vi "Main.vi"(8 "error in":errorcluster, 11 "Head_ScopeSim in":refnum<class "Head_ScopeSim.lvclass">) -> (0 "error out":errorcluster, 3 "Head_ScopeSim out":refnum<class "Head_ScopeSim.lvclass">)   [LabVIEW 2019, in "Head_ScopeSim.lvclass"]
doc: "The <b>Queued Message Handler</b> of the Worker that owns this VI."
uses:
  Head_ScopeSim.lvclass
  C:/Program Files (x86)/National Instruments/LabVIEW 2019/vi.lib/addons/_Workers/Library/Classes/Worker/Worker.lvclass
  Head_ScopeSim.lvclass/Head_ScopeSim.ctl
  Initialization Data.ctl
  Response Cases.ctl
  rql_Create gRPC Server.ctl
  gRPC Server/gRPC Server/rwr_Create gRPC Server.ctl
  rql_Destroy gRPC Server.ctl
  Scope Simulator/rqp_Scope Configuration.ctl
  Scope Simulator/rqp_Run Scope.ctl
  gRPC Server/gRPC Server/rqp_Msg_ToClient_2.ctl
  Generated_server/RPC Messages/w4lvgrpc_Msg_ToClient_2.ctl
  gRPC Server/gRPC Server/rqp_Msg_ToClient_3.ctl
  Generated_server/RPC Messages/w4lvgrpc_Msg_ToClient_3.ctl
  Generated_server/RPC Messages/w4lvgrpc_State.ctl
  <vilib>/addons/_Workers/Library/Classes/Message Queue/Message Queue.lvclass
  Scope Simulator/Scope Simulator.lvclass
  gRPC Server/gRPC Server/gRPC Server.lvclass
  Generated_server/Generated_server.lvlib
panel:
  out "Client ID":u64
  out "Client Connected":bool
  out "Listening Port":i32
  out "Server Listening":bool
  in  "Server Address":string="localhost:50070"
  in  "Destroy gRPC Server":bool
  in  "Create gRPC Server":bool
  # "Workers <-> Python gRPC Example"
  # "Scope Simulator"
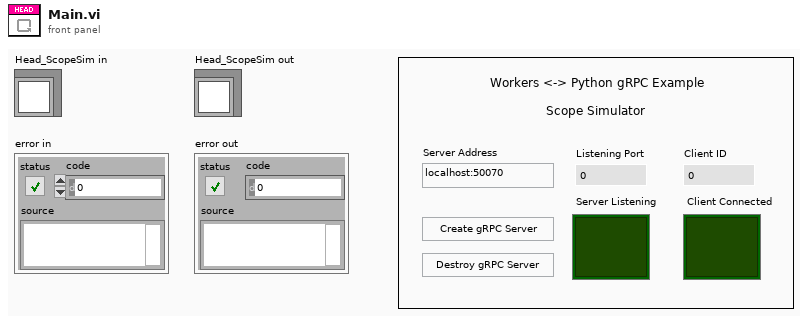
[diagram p1: front panel]
types:
  T1 = typedef "Head_ScopeSim.lvclass/Initialization Data.ctl" = cluster{"Response Cases":T2}
  T2 = typedef "Head_ScopeSim.lvclass/Response Cases.ctl" = cluster{"Placeholder - Can be deleted":string}
  T3 = typedef "Head_ScopeSim.lvclass/rql_Create gRPC Server.ctl" = cluster{"String":string}
  T4 = typedef "gRPC Server (scope.proto).lvlib/gRPC Server.lvclass/rwr_Create gRPC Server.ctl" = cluster{"Server Key File (.key)":path, "Server Certificate File (.crt)":path, "Server Address":string}
  T5 = typedef "Head_ScopeSim.lvclass/rql_Destroy gRPC Server.ctl" = cluster{"String":string}
  T6 = typedef "Scope Simulator.lvclass/rqp_Scope Configuration.ctl" = cluster{"physical_channel":string, "sample_rate_hz":dbl, "samples_per_read":i32}
  T7 = typedef "Scope Simulator.lvclass/rqp_Run Scope.ctl" = cluster{"Run Scope ?":bool}
  T8 = typedef "gRPC Server (scope.proto).lvlib/gRPC Server.lvclass/rqp_Msg_ToClient_2.ctl" = cluster{"w4lvgrpc_Msg_ToClient_2":T9}
  T9 = typedef "Generated_server.lvlib/w4lvgrpc_Msg_ToClient_2.ctl" = cluster{"y":dbl[], "dt":dbl, "t0":dbl, "label":string, "acquisitions":i32}
  T10 = typedef "gRPC Server (scope.proto).lvlib/gRPC Server.lvclass/rqp_Msg_ToClient_3.ctl" = cluster{"w4lvgrpc_Msg_ToClient_3":T11}
  T11 = typedef "Generated_server.lvlib/w4lvgrpc_Msg_ToClient_3.ctl" = cluster{"state":T12}
  T12 = typedef "Generated_server.lvlib/w4lvgrpc_State.ctl" = enum32{"STOPPED", "RUNNING", "ERROR"}
  T13 = typedef "gRPC Server (scope.proto).lvlib/gRPC Server.lvclass/rwr_Create gRPC Server Reply.ctl" = cluster{"Listening Port":i32}
  T14 = typedef "gRPC Server (scope.proto).lvlib/gRPC Server.lvclass/rsp_Connection Notify.ctl" = cluster{"gRPC ID":T15, "Connected?":bool}
  T15 = typedef "grpc-lvsupport-release.lvlib/grpcId.ctl" = u64
  T16 = typedef "gRPC Server (scope.proto).lvlib/gRPC Server.lvclass/rsp_Server Error.ctl" = errorcluster
  T17 = typedef "gRPC Server (scope.proto).lvlib/gRPC Server.lvclass/rsp_Msg_ToServer_1.ctl" = cluster{"w4lvgrpc_Msg_ToServer_1":T18}
  T18 = typedef "Generated_server.lvlib/w4lvgrpc_Msg_ToServer_1.ctl" = cluster{"physical_channel":string, "sample_rate_hz":dbl, "samples_per_read":i32}
  T19 = typedef "gRPC Server (scope.proto).lvlib/gRPC Server.lvclass/rsp_Msg_ToServer_2.ctl" = cluster{"w4lvgrpc_Msg_ToServer_2":T20}
  T20 = typedef "Generated_server.lvlib/w4lvgrpc_Msg_ToServer_2.ctl" = cluster{"run":bool}
  T21 = typedef "Scope Simulator.lvclass/rsp_Generated Waveform.ctl" = cluster{"y":dbl[], "Acquisitions":i32}
  T22 = typedef "Scope Simulator.lvclass/rsp_Scope Status.ctl" = enum32{"STOPPED", "RUNNING", "ERROR"}
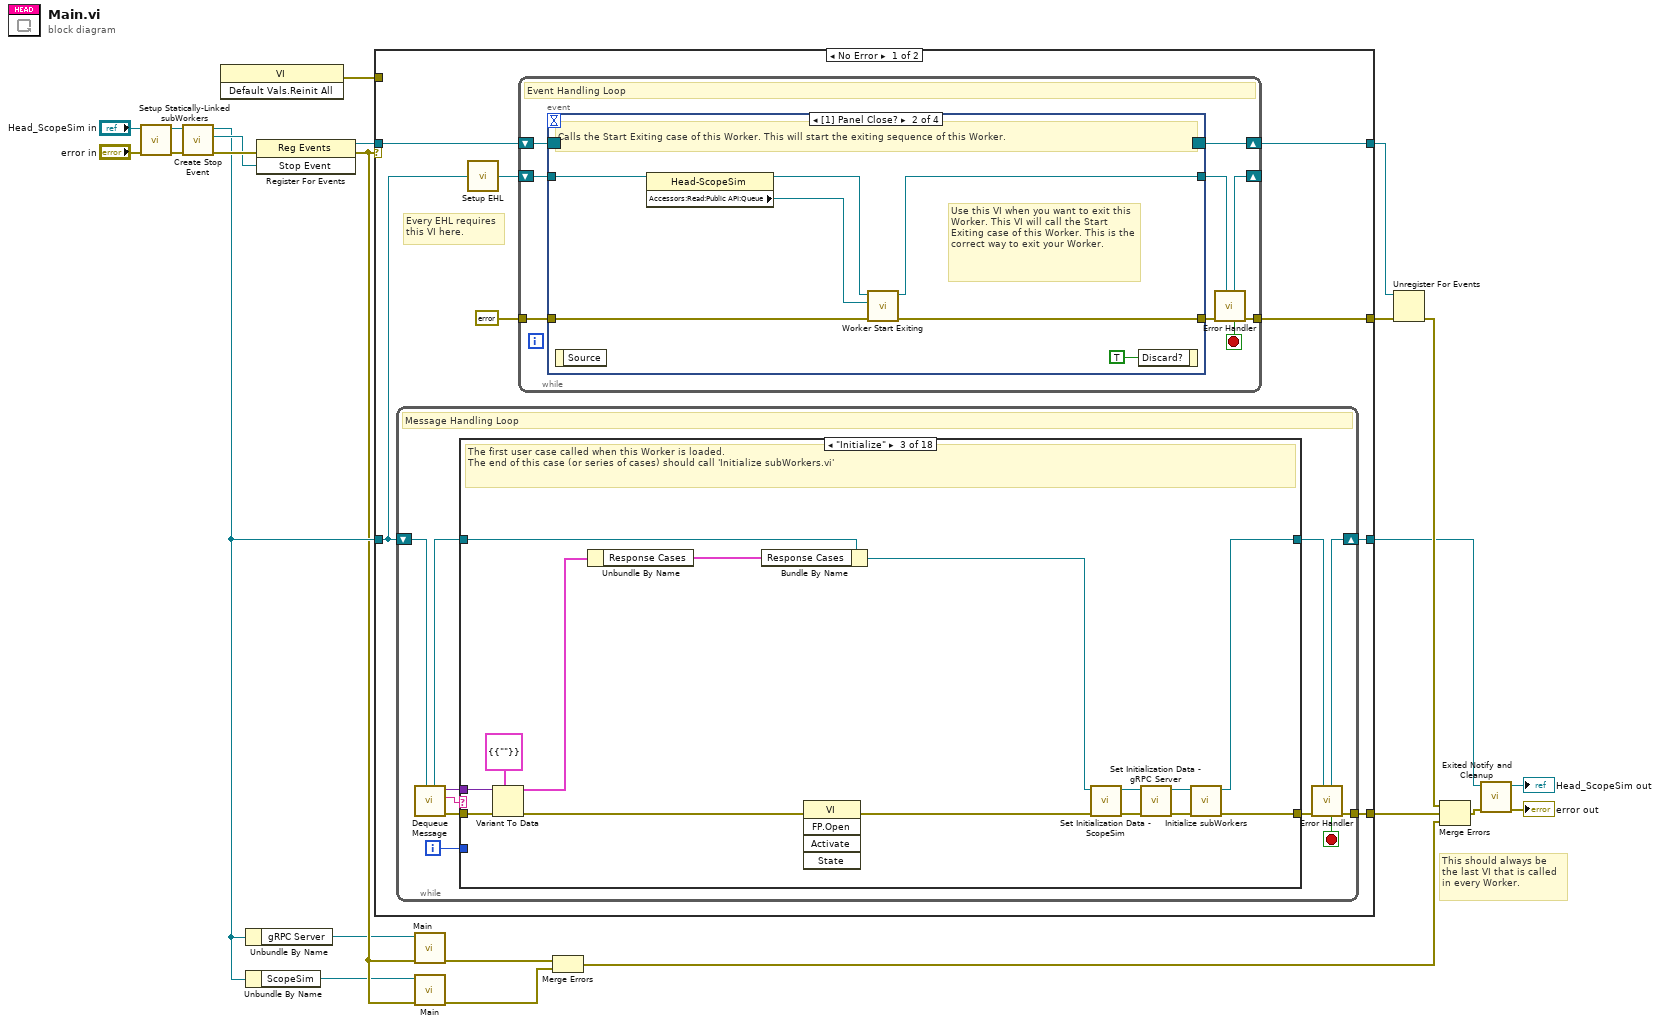
[diagram p0: block diagram]
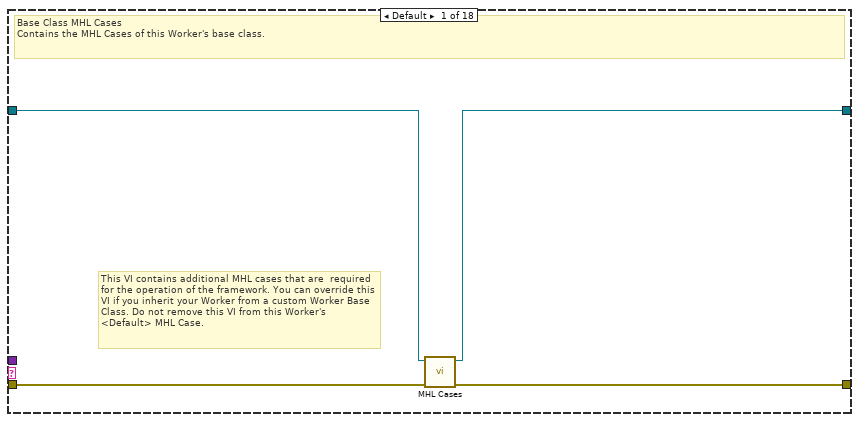
[diagram p2: hidden frame]
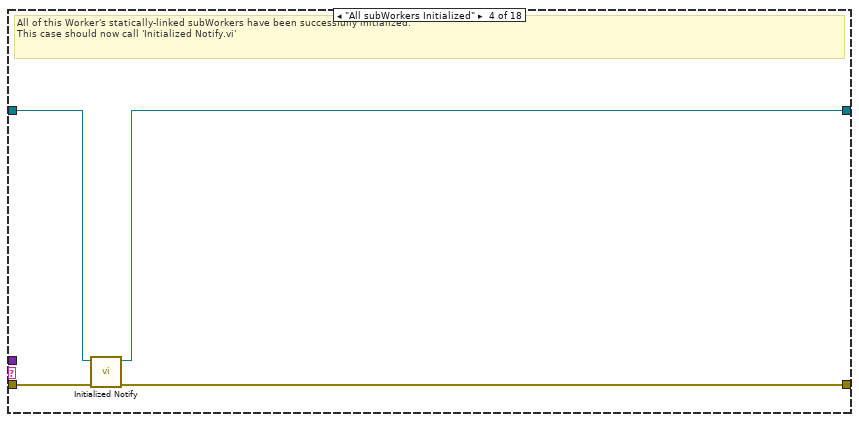
[diagram p4: hidden frame]
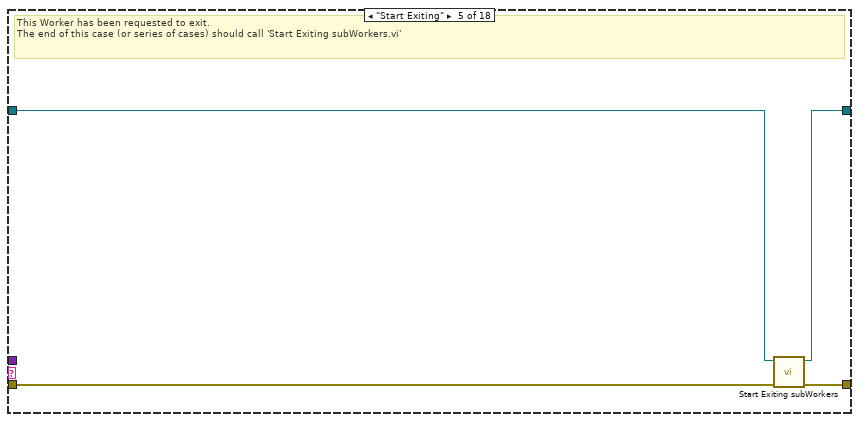
[diagram p5: hidden frame]
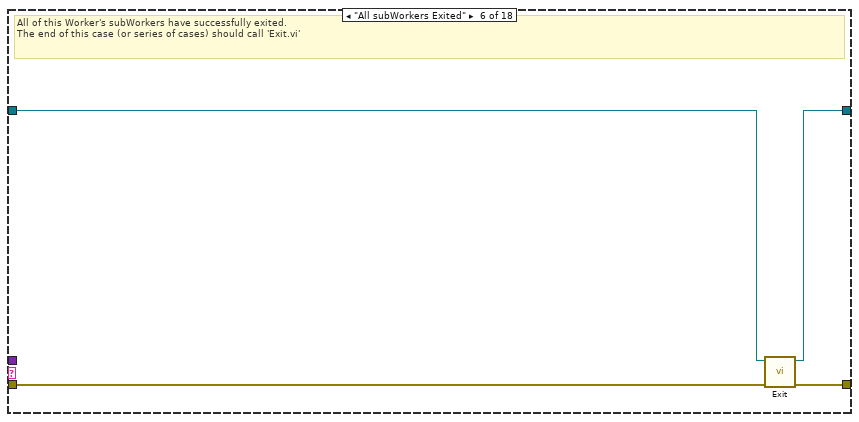
[diagram p6: hidden frame]
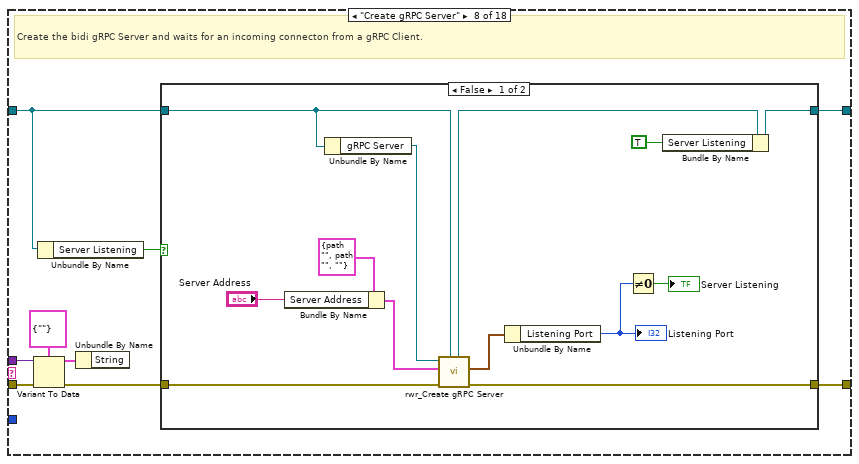
[diagram p8: hidden frame]
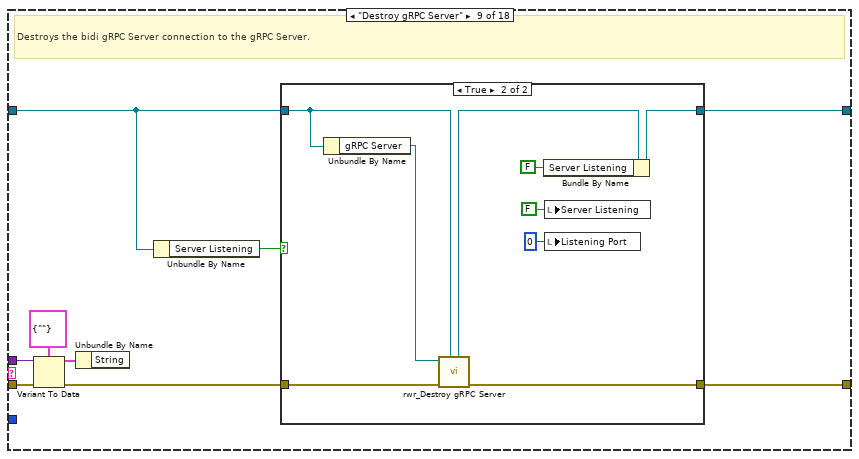
[diagram p10: hidden frame]
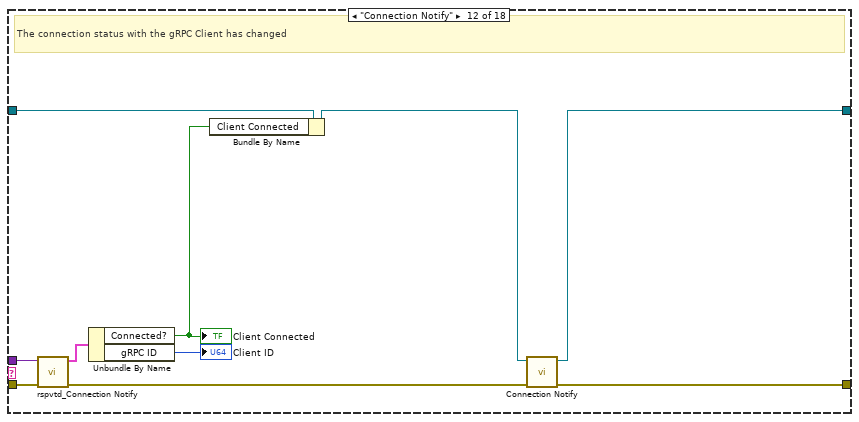
[diagram p14: hidden frame]
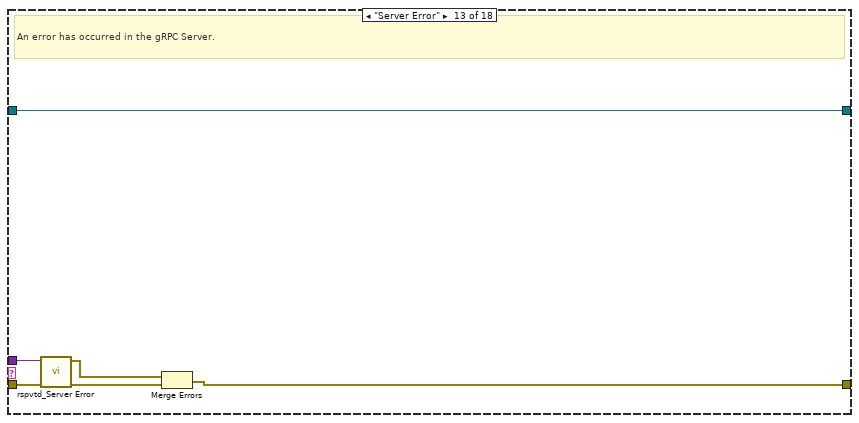
[diagram p15: hidden frame]
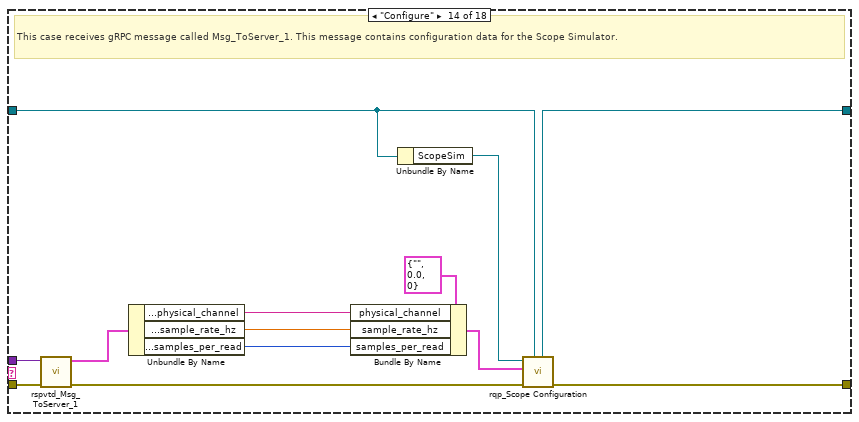
[diagram p16: hidden frame]
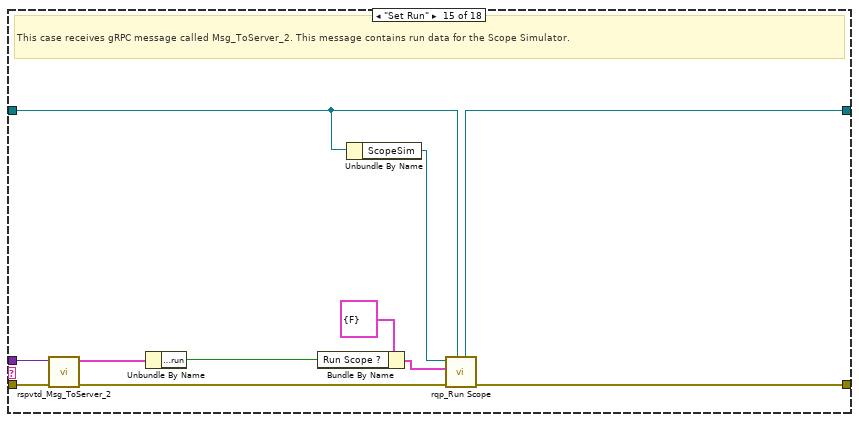
[diagram p17: hidden frame]
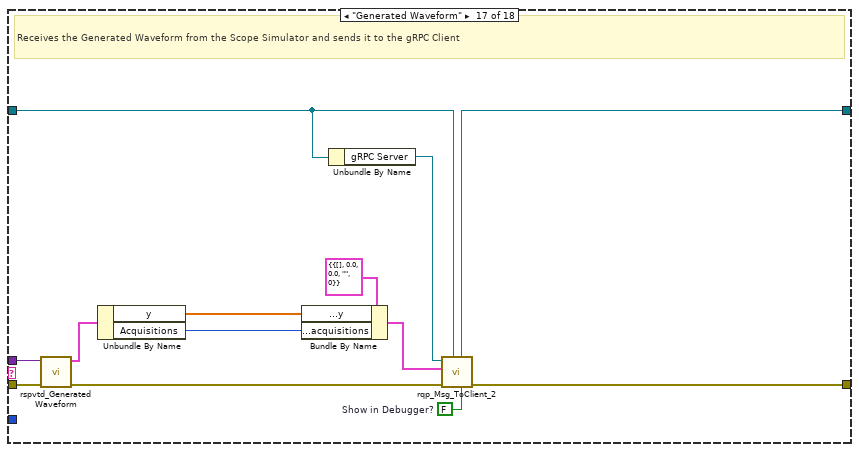
[diagram p19: hidden frame]
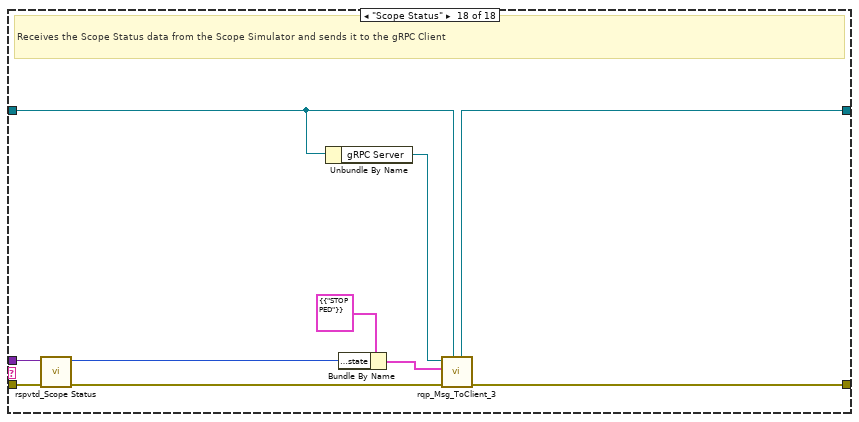
[diagram p20: hidden frame]
diagram:
  # "This should always be the last VI that is called in every Worker."
  n1 = call "Setup Statically-Linked subWorkers.vi"("error in"="error in", "Head_ScopeSim in"="Head_ScopeSim in") -> ("error out"=w9:errorcluster, "Head_ScopeSim out"=w7:refnum<class "Head_ScopeSim.lvclass">)  [unwired: 8 in]
  n2 = call-dynamic "Create Stop Event.vi"("error in"=w9, "Worker"=w7) -> ("error out"=w18:errorcluster, "Stop Event"=w15:refnum<user-event>, "Worker out"=w12:refnum<class "Head_ScopeSim.lvclass">)  [unwired: 7 in]
  n3 = invoke class="VI" method="Default Vals.Reinit All"() -> (error out=w3:errorcluster)  [unwired: 3 in, 2 out]
  n4 = Unbundle By Name(w12) -> ("gRPC Server"=w4:refnum<class "gRPC Server.lvclass">)
  n5 = Unbundle By Name(w12) -> ("ScopeSim"=w1:refnum<class "Scope Simulator.lvclass">)
  n6 = register-events(error in=w18, w15) -> (reference out=w17:refnum<event-registration>, error out=w10:errorcluster)  [unwired: 1 in]
  n7 = case shown="No Error" w10 {
    tunnel: w12 -> [w26 w221]
    tunnel: [w24 w222] -> w16
    tunnel: w17 -> [w31 w223]
    tunnel: [w28 w224] -> w22
    tunnel: [w30 w223] -> w21
    tunnel: [w25 w220] -> w19
    selector: w10 -> [_ w224]
    tunnel: w3 -> [_ _]
    frame No Error {
      # "Every EHL requires\nthis VI here."
      n8 = while {
        shift-right: [w40] -> w25
        shift-left: w26 -> [w42]
        tunnel: [w41] -> w24
        i -> [w33]
        stop <- w34 stop-if-true
        # "Message Handling Loop"
        n9 = call-dynamic "Dequeue Message.vi"("Worker"=w42) -> ("error out"=w39:errorcluster, "Case out"=w35:string, "Data out"=w32:variant, "Worker out"=w37:refnum<class "Head_ScopeSim.lvclass">)  [unwired: 6 in, 1 out]
        n10 = case "Worker MHL Case Structure (DO NOT CHANGE LABEL NAME)" shown="\"Initialize\"" w35 {
          tunnel: w39 -> [w46 w47 w61 w66 w68 w75 w77 w86 w110 w123 w125 w135 w141 w154 w165 w167 w180 w190]
          tunnel: [w45 w47 w63 w64 w71 w74 w77 w81 w105 w123 w125 w128 w137 w150 w161 w167 w177 w187] -> w38
          tunnel: w37 -> [w44 w48 w60 w67 w69 w73 w76 w79 w103 w122 w124 w134 w140 w148 w159 w166 w175 w185]
          tunnel: [w43 w48 w62 w65 w70 w72 w76 w80 w104 w122 w124 w130 w140 w149 w160 w166 w176 w186] -> w36
          tunnel: w33 -> [_ _ _ _ _ _ _ _ _ _ _ _ _ _ _ _ _ _]
          tunnel: w32 -> [_ _ w59 _ _ _ _ w83 w107 _ _ w133 w138 w152 w164 _ w178 w188]
          frame Default {
            # "This VI contains additional MHL cases that are  required for the operation of the framework. You can override this VI if you inherit your Worker from a custom Worker Base Class. Do not remove this VI from this Worker's <Default> MHL Case."
            # "Base Class MHL Cases\nContains the MHL Cases of this Worker's base class."
            n11 = call-dynamic "MHL Cases.vi"("error in"=w46, "Worker in"=w44) -> ("error out"=w45:errorcluster, "Worker out"=w43:refnum<class "Head_ScopeSim.lvclass">)  [unwired: 8 in]
          }
          frame "------------ FRAMEWORK CASES -----------" {
            # "Start of Workers Framework Cases"
          }
          frame "Initialize" {
            # "The first user case called when this Worker is loaded.\nThe end of this case (or series of cases) should call 'Initialize subWorkers.vi'"
            n12 = Variant To Data(error in=w61, type=T1 {"Response Cases"={"Placeholder - Can be deleted"=""}} ("Initialization Data"), Variant=w59) -> (data=w58:T1, error out=w50:errorcluster)
            n13 = Unbundle By Name(w58) -> ("Response Cases"=w57:T2)
            n14 = Bundle By Name(cluster=w60, "Response Cases"=w57) -> (w52:refnum<class "Head_ScopeSim.lvclass">)
            n15 = invoke class="VI" method="FP.Open"(error in=w50) -> (error out=w49:errorcluster)  [unwired: 4 in, 4 out]
            n16 = call "Set Initialization Data - ScopeSim.vi"("error in"=w49, "Head_ScopeSim in"=w52) -> ("error out"=w53:errorcluster, "Head_ScopeSim out"=w51:refnum<class "Head_ScopeSim.lvclass">)  [unwired: 8 in]
            n17 = call "Set Initialization Data - gRPC Server.vi"("error in"=w53, "Head_ScopeSim in"=w51) -> ("error out"=w55:errorcluster, "Head_ScopeSim out"=w54:refnum<class "Head_ScopeSim.lvclass">)  [unwired: 8 in]
            n18 = call-dynamic "Initialize subWorkers.vi"("error in"=w55, "Worker"=w54) -> ("error out"=w63:errorcluster, "dup Worker out"=w62:refnum<class "Head_ScopeSim.lvclass">)  [unwired: 8 in]
          }
          frame "All subWorkers Initialized" {
            # "All of this Worker's statically-linked subWorkers have been successfully initialized.\nThis case should now call 'Initialized Notify.vi'"
            n19 = call-dynamic "Initialized Notify.vi"("error in"=w66, "Worker"=w67) -> ("error out"=w64:errorcluster, "dup Worker out"=w65:refnum<class "Head_ScopeSim.lvclass">)  [unwired: 8 in]
          }
          frame "Start Exiting" {
            # "This Worker has been requested to exit. \nThe end of this case (or series of cases) should call 'Start Exiting subWorkers.vi'"
            n20 = call-dynamic "Start Exiting subWorkers.vi"("error_in"=w68, "Worker"=w69) -> ("error out"=w71:errorcluster, "dup Worker out"=w70:refnum<class "Head_ScopeSim.lvclass">)  [unwired: 8 in]
          }
          frame "All subWorkers Exited" {
            # "All of this Worker's subWorkers have successfully exited. \nThe end of this case (or series of cases) should call 'Exit.vi'"
            n21 = call-dynamic "Exit.vi"("error_in"=w75, "Worker"=w73) -> ("error out"=w74:errorcluster, "dup Worker out"=w72:refnum<class "Head_ScopeSim.lvclass">)  [unwired: 8 in]
          }
          frame "------------- LOCAL API CASES -------------" {
            # "Start of Workers Local API Cases"
          }
          frame "Create gRPC Server" {
            # "Create the bidi gRPC Server and waits for an incoming connecton from a gRPC Client."
            n22 = Variant To Data(error in=w86, type=T3 {"String"=""} ("Data"), Variant=w83) -> (data=w82:T3, error out=w85:errorcluster)
            n23 = Unbundle By Name(w79) -> ("Server Listening"=w78:bool)
            n24 = Unbundle By Name(w82) -> ()  [unwired: 1 out]
            n25 = case shown="False" w78 {
              tunnel: w85 -> [w99 w100]
              tunnel: [w98 w100] -> w81
              tunnel: [w88 w101] -> w80
              tunnel: w79 -> [w96 w101]
              frame False {
                n26 = Bundle By Name(cluster=T4 {"Server Key File (.key)"=path "", "Server Certificate File (.crt)"=path "", "Server Address"=""} ("Data in"), "Server Address"="Server Address") -> (w93:T4)
                n27 = Unbundle By Name(w96) -> ("gRPC Server"=w95:refnum<class "gRPC Server.lvclass">)
                n28 = call "rwr_Create gRPC Server.vi"("Caller in"=w96, "error in"=w99, "Data in"=w93, "gRPC Server in"=w95) -> ("error out"=w98:errorcluster, "Reply Data out"=w91:T13, "dup Caller out"=w97:refnum<class "Head_ScopeSim.lvclass">)  [unwired: 4 in, 1 out]
                n29 = Unbundle By Name(w91) -> ("Listening Port"=w90:i32)
                "Listening Port" <- w90
                n30 = Not Equal To 0?(x=w90) -> (x != 0?=→"Server Listening":bool)
                n31 = Bundle By Name(cluster=w97, "Server Listening"=TRUE) -> (w88:refnum<class "Head_ScopeSim.lvclass">)
              }
              frame True {
                # "Already listening. Nothing to do."
              }
            }
          }
          frame "Destroy gRPC Server" {
            # "Destroys the bidi gRPC Server connection to the gRPC Server."
            n32 = Variant To Data(error in=w110, type=T5 {"String"=""} ("Data"), Variant=w107) -> (data=w106:T5, error out=w109:errorcluster)
            n33 = Unbundle By Name(w106) -> ()  [unwired: 1 out]
            n34 = Unbundle By Name(w103) -> ("Server Listening"=w102:bool)
            n35 = case shown="True" w102 {
              tunnel: w109 -> [w111 w121]
              tunnel: [w111 w116] -> w105
              tunnel: [w112 w117] -> w104
              tunnel: w103 -> [w112 w119]
              frame False {
                # "Server not listening. Nothing to do"
              }
              frame True {
                n36 = Unbundle By Name(w119) -> ("gRPC Server"=w118:refnum<class "gRPC Server.lvclass">)
                n37 = call "rwr_Destroy gRPC Server.vi"("Caller in"=w119, "error in"=w121, "gRPC Server in"=w118) -> ("error out"=w116:errorcluster, "dup Caller out"=w120:refnum<class "Head_ScopeSim.lvclass">)  [unwired: 5 in, 2 out]
                n38 = Bundle By Name(cluster=w120, "Server Listening"=FALSE) -> (w117:refnum<class "Head_ScopeSim.lvclass">)
                n39 = local write "Server Listening"(FALSE ("Server Listening")) -> ()
                n40 = local write "Listening Port"(0 ("Listening Port")) -> ()
              }
            }
          }
          frame "------------- RESPONSE CASES --------------" {
            # "Start of Workers Response Cases"
          }
          frame "~~~~~~~~ gRPC Server ~~~~~~~~~~~~" {
          }
          frame "Connection Notify" {
            # "The connection status with the gRPC Client has changed"
            n41 = call "rspvtd_Connection Notify.vi"("error in"=w135, "Data in"=w133) -> ("error out"=w129:errorcluster, "Data out"=w132:T14)  [unwired: 8 in]
            n42 = Unbundle By Name(w132) -> ("Connected?"=w127:bool, "gRPC ID"=→"Client ID":T15)
            "Client Connected" <- w127
            n43 = Bundle By Name(cluster=w134, "Client Connected"=w127) -> (w131:refnum<class "Head_ScopeSim.lvclass">)
            n44 = call "Connection Notify.vi"("error in (no error)"=w129, "Head_ScopeSim in"=w131) -> ("error out"=w128:errorcluster, "Head_ScopeSim out"=w130:refnum<class "Head_ScopeSim.lvclass">)  [unwired: 8 in]
          }
          frame "Server Error" {
            # "An error has occurred in the gRPC Server."
            n45 = call "rspvtd_Server Error.vi"("error in"=w141, "Data in"=w138) -> ("error out"=w139:errorcluster, "Data out"=w136:T16)  [unwired: 8 in]
            n46 = Merge Errors(w136, w139) -> (w137:errorcluster)
          }
          frame "Configure" {
            # "This case receives gRPC message called Msg_ToServer_1. This message contains configuration data for the Scope Simulator."
            n47 = call "rspvtd_Msg_ToServer_1.vi"("error in"=w154, "Data in"=w152) -> ("error out"=w153:errorcluster, "Data out"=w151:T17)  [unwired: 8 in]
            n48 = Unbundle By Name(w151) -> ("w4lvgrpc_Msg_ToServer_1.physical_channel"=w142:string, "w4lvgrpc_Msg_ToServer_1.sample_rate_hz"=w143:dbl, "w4lvgrpc_Msg_ToServer_1.samples_per_read"=w144:i32)
            n49 = Bundle By Name(cluster=T6 {"physical_channel"="", "sample_rate_hz"=0.0, "samples_per_read"=0} ("Data in"), "physical_channel"=w142, "sample_rate_hz"=w143, "samples_per_read"=w144) -> (w145:T6)
            n50 = Unbundle By Name(w148) -> ("ScopeSim"=w147:refnum<class "Scope Simulator.lvclass">)
            n51 = call "rqp_Scope Configuration.vi"("Caller in"=w148, "error in"=w153, "Data in"=w145, "Scope Simulator in"=w147) -> ("error out"=w150:errorcluster, "dup Caller out"=w149:refnum<class "Head_ScopeSim.lvclass">)  [unwired: 5 in, 1 out]
          }
          frame "Set Run" {
            # "This case receives gRPC message called Msg_ToServer_2. This message contains run data for the Scope Simulator."
            n52 = call "rspvtd_Msg_ToServer_2.vi"("error in"=w165, "Data in"=w164) -> ("error out"=w162:errorcluster, "Data out"=w163:T19)  [unwired: 8 in]
            n53 = Unbundle By Name(w163) -> ("w4lvgrpc_Msg_ToServer_2.run"=w155:bool)
            n54 = Bundle By Name(cluster=T7 {"Run Scope ?"=FALSE} ("Data in"), "Run Scope ?"=w155) -> (w156:T7)
            n55 = Unbundle By Name(w159) -> ("ScopeSim"=w158:refnum<class "Scope Simulator.lvclass">)
            n56 = call "rqp_Run Scope.vi"("Caller in"=w159, "error in"=w162, "Data in"=w156, "Scope Simulator in"=w158) -> ("error out"=w161:errorcluster, "dup Caller out"=w160:refnum<class "Head_ScopeSim.lvclass">)  [unwired: 5 in, 1 out]
          }
          frame "~~~~~~~~ Scope Simulator ~~~~~~~~~" {
          }
          frame "Generated Waveform" {
            w168 = FALSE  # Show in Debugger?
            # "Receives the Generated Waveform from the Scope Simulator and sends it to the gRPC Client"
            n57 = call "rspvtd_Generated Waveform.vi"("error in"=w180, "Data in"=w178) -> ("error out"=w179:errorcluster, "Data out"=w173:T21)  [unwired: 8 in]
            n58 = Unbundle By Name(w173) -> ("y"=w170:dbl[], "Acquisitions"=w169:i32)
            n59 = Bundle By Name(cluster=T8 {"w4lvgrpc_Msg_ToClient_2"={"y"=[], "dt"=0.0, "t0"=0.0, "label"="", "acquisitions"=0}} ("Data in"), "w4lvgrpc_Msg_ToClient_2.y"=w170, "w4lvgrpc_Msg_ToClient_2.acquisitions"=w169) -> (w171:T8)
            n60 = Unbundle By Name(w175) -> ("gRPC Server"=w174:refnum<class "gRPC Server.lvclass">)
            n61 = call "rqp_Msg_ToClient_2.vi"("Show in Debugger?"=w168, "Caller in"=w175, "error in"=w179, "Data in"=w171, "gRPC Server in"=w174) -> ("error out"=w177:errorcluster, "dup Caller out"=w176:refnum<class "Head_ScopeSim.lvclass">)  [unwired: 4 in, 1 out]
          }
          frame "Scope Status" {
            # "Receives the Scope Status data from the Scope Simulator and sends it to the gRPC Client"
            n62 = call "rspvtd_Scope Status.vi"("error in"=w190, "Data in"=w188) -> ("error out"=w189:errorcluster, "Data out"=w181:T22)  [unwired: 8 in]
            n63 = Unbundle By Name(w185) -> ("gRPC Server"=w184:refnum<class "gRPC Server.lvclass">)
            n64 = Bundle By Name(cluster=T10 {"w4lvgrpc_Msg_ToClient_3"={"state"=enum."STOPPED"}} ("Data in"), "w4lvgrpc_Msg_ToClient_3.state"=w181) -> (w182:T10)
            n65 = call "rqp_Msg_ToClient_3.vi"("Caller in"=w185, "error in"=w189, "Data in"=w182, "gRPC Server in"=w184) -> ("error out"=w187:errorcluster, "dup Caller out"=w186:refnum<class "Head_ScopeSim.lvclass">)  [unwired: 5 in, 1 out]
          }
        }
        n66 = call-dynamic "Error Handler.vi"("Worker"=w36, "error_in"=w38) -> ("error out"=w41:errorcluster, "Stop Loop"=w34:bool, "Worker out"=w40:refnum<class "Head_ScopeSim.lvclass">)  [unwired: 7 in]
      }
      n67 = call-dynamic "Setup EHL.vi"("Worker"=w26) -> ("Worker out"=w27:refnum<class "Head_ScopeSim.lvclass">)  [unwired: 14 in]
      n68 = while "Event Handling Loop" {
        shift-right: [w199] -> w30
        shift-left: w31 -> [w198]
        tunnel: [w194] -> w28
        tunnel: errorcluster {"status"=FALSE, "code"=0, "source"=""} ("error constant") -> [w196]
        shift-right: [w192] -> _
        shift-left: w27 -> [w197]
        stop <- w191 stop-if-true
        # "Event Handling Loop"
        n69 = event shown="[1] Panel Close?" {
          selector: w198 -> [_ _ _ _]
          dyn-events: [_ _ _ _] -> w199
          timeout: _ -> [_ _ _ _]
          tunnel: [w203 w210 w214 w218] -> w195
          tunnel: w196 -> [w204 w209 w215 w219]
          tunnel: w197 -> [w202 w208 w213 w217]
          tunnel: [w201 w207 w212 w216] -> w193
          event User Event {
            # "This case and its contents must always be included in every EHL that you use, so that the framework can automatically stop the EHL."
            # "EHL Stop Event. This EHL exits from this case."
            n70 = event-data() -> ("Stop Event Data"=w200:variant)  [unwired: 1 in]
            n71 = call-dynamic "EHL Stop - EHL Case.vi"("error in"=w204, "Stop Event Data"=w200, "Worker"=w202) -> ("error out"=w203:errorcluster, "Worker out"=w201:refnum<class "Head_ScopeSim.lvclass">)  [unwired: 7 in]
          }
          event Panel Close? {
            # "Use this VI when you want to exit this Worker. This VI will call the Start Exiting case of this Worker. This is the correct way to exit your Worker."
            # "Calls the Start Exiting case of this Worker. This will start the exiting sequence of this Worker."
            n72 = event-data() -> ()  [unwired: 1 in, 1 out]
            n73 = property class="Head-ScopeSim"(reference=w208) -> (reference out=w206:refnum<class "Head_ScopeSim.lvclass">, "Accessors:Read:Public API:Queue"=w205:refnum<class "Message Queue.lvclass">)  [unwired: 1 in, 1 out]
            n74 = call-dynamic "Worker Start Exiting.vi"("error_in"=w209, "Message Queue"=w205, "Worker"=w206) -> ("error out"=w210:errorcluster, "dup Worker out"=w207:refnum<class "Head_ScopeSim.lvclass">)  [unwired: 7 in]
            n75 = event-data ("Event Filter Node")("Discard?"=TRUE) -> ()  [unwired: 1 in, 1 out]
          }
          event "Create gRPC Server": Value Change {
            n76 = event-data() -> ()  [unwired: 1 in, 1 out]
            n77 = call "rql_Create gRPC Server.vi"("error in"=w215, "Head_ScopeSim in"=w213) -> ("error out"=w214:errorcluster, "dup Head_ScopeSim out"=w212:refnum<class "Head_ScopeSim.lvclass">)  [unwired: 8 in]
          }
          event "Destroy gRPC Server": Value Change {
            n78 = event-data() -> ()  [unwired: 1 in, 1 out]
            n79 = call "rql_Destroy gRPC Server.vi"("error in"=w219, "Head_ScopeSim in"=w217) -> ("error out"=w218:errorcluster, "dup Head_ScopeSim out"=w216:refnum<class "Head_ScopeSim.lvclass">)  [unwired: 8 in]
          }
        }
        n80 = call-dynamic "Error Handler.vi"("Worker"=w193, "error_in"=w195) -> ("error out"=w194:errorcluster, "Stop Loop"=w191:bool, "Worker out"=w192:refnum<class "Head_ScopeSim.lvclass">)  [unwired: 7 in]
      }
    }
    frame Error {
      n81 = call-dynamic "Error Handler.vi"("Worker"=w221, "error_in"=w224) -> ("error out"=w222:errorcluster, "Worker out"=w220:refnum<class "Head_ScopeSim.lvclass">)  [unwired: 7 in, 1 out]
    }
  }
  n82 = call-dynamic "Main.vi"("error in"=w10, "gRPC Server in"=w4) -> ("error out"=w6:errorcluster)  [unwired: 8 in, 1 out]
  n83 = call-dynamic "Main.vi"("error in"=w10, "Scope Simulator in"=w1) -> ("error out"=w2:errorcluster)  [unwired: 8 in, 1 out]
  n84 = Merge Errors(w6, w2) -> (w5:errorcluster)
  n85 = Unregister For Events(event registration refnum=w21, error in=w22) -> (error out=w23:errorcluster)
  n86 = Merge Errors(w23, w16, w5) -> (w20:errorcluster)
  n87 = call-dynamic "Exited Notify and Cleanup.vi"("error_in"=w20, "Worker"=w19) -> ("error out"=→"error out":errorcluster, "dup Worker out"=→"Head_ScopeSim out":refnum<class "Head_ScopeSim.lvclass">)  [unwired: 8 in]
